vi "NicmosFilterControl.vi"(2 "Initialize":bool, 7 "FILTER":T1, 9 "error in (no error)":errorcluster caption="entrée d'erreur") -> (6 "error out":errorcluster caption="sortie d'erreur")   [LabVIEW 2009]
uses:
  Controls/NICMOS.FILTER.ctl
  <vilib>/Utility/config.llb/Write Key (String).vi
  NicmosGlobal.vi
  <vilib>/Utility/config.llb/NI_LVConfig.lvlib
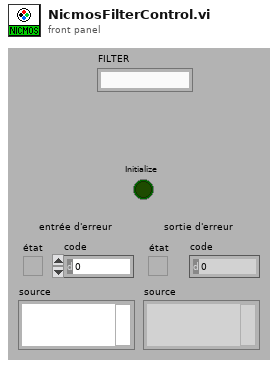
[diagram p1: front panel]
types:
  T1 = typedef "NICMOS.FILTER.ctl" = string
  T2 = typedef "NICMOS.FILTERLIST.ctl" = T1[]
  T3 = typedef "NI_LVConfig.lvlib/Config Data RefNum.ctl" = refnum<k1>
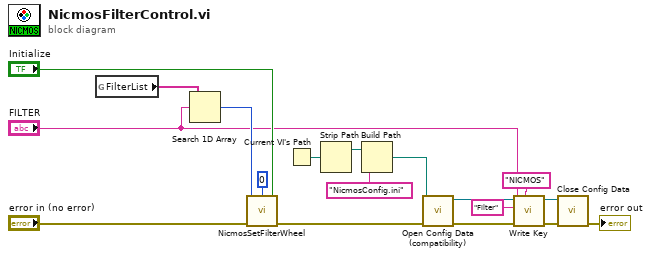
[diagram p0: block diagram]
diagram:
  n1 = global read "NicmosGlobal.vi" "FilterList"() -> (w3:T2)
  n2 = Search 1D Array(1D array=w3, element="FILTER") -> (index of element=w2:i32)  [unwired: 1 in]
  n3 = call "NicmosSetFilterWheel.vi"("error in (no error)"="error in (no error)", "Filter"=w2, "Offset"=i16 0, "Initialize"="Initialize") -> ("error out"=w5:errorcluster)  [unwired: 3 in]
  n4 = Current VI's Path() -> (path=w15:path)
  n5 = Strip Path(path=w15) -> (stripped path=w4:path)  [unwired: 1 out]
  n6 = Build Path(base path=w4, name or relative path="NicmosConfig.ini" ("nom ou chemin relatif")) -> (appended path=w13:path)
  n7 = call <vilib>:"Open Config Data (compatibility).vi"("error in (no error)"=w5, "configuration file path"=w13) -> ("error out"=w12:errorcluster, "refnum"=w11:T3)  [unwired: 7 in, 1 out]
  n8 = call-poly <vilib>:"Write Key.vi"("section"="NICMOS", "error in (no error)"=w12, "value"="FILTER", "key"="Filter", "refnum"=w11) -> ("error out"=w8:errorcluster, "refnum out"=w7:T3)  [unwired: 4 in, 1 out]
  n9 = call <vilib>:"Close Config Data.vi"("error in (no error)"=w8, "refnum"=w7) -> ("error out"=→"error out":errorcluster)  [unwired: 8 in, 1 out]
